vi "Configure.vi"(8 "error in (no error)":errorcluster, 11 "Template in":refnum<class "BMC.lvclass">) -> (0 "error out":errorcluster, 2 "cancelled?":bool, 3 "Template out":refnum<class "BMC.lvclass">)   [LabVIEW 2012, in "BMC.lvclass"]
doc: "The configure method configures the details for the RabbitMQ connection. \n\nIn the derived class, make a call to the parent for setting these parameters."
uses:
  BMC.lvclass
  <vilib>/Utility/miscctls.llb/LVPointTypeDef.ctl
  BMC.lvclass/BMC.ctl
  <vilib>/Distrio/Murmex/Murmex/Murmex.lvclass
panel:
  in  "Mapping file":path=path "D:/CLSM_Project/BMC/MultiMap.txt"
  in  "Flat mirror file":path=path "D:/CLSM_Project/BMC/zerovolt.txt"
  in  "button:call parent":bool
  in  "button:ok":bool
  in  "button:cancel":bool
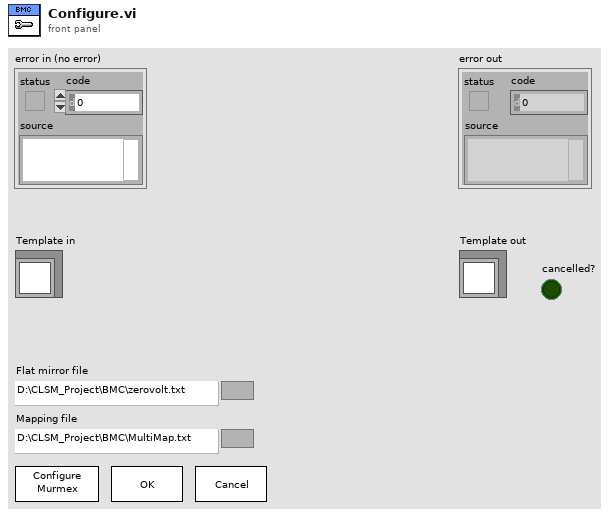
[diagram p1: front panel]
types:
  T1 = typedef "LVPointTypeDef.ctl" = cluster{"Horizontal":i16, "Vertical":i16}
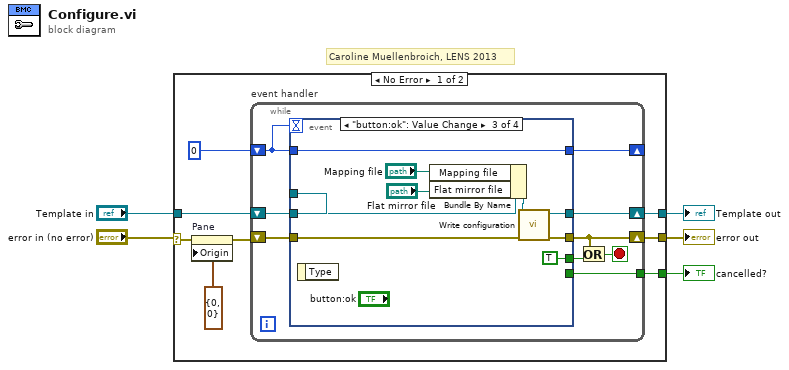
[diagram p0: block diagram]
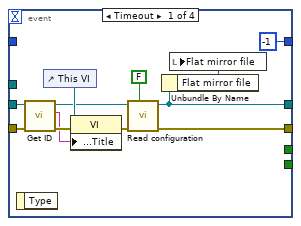
[diagram p2: hidden frame]
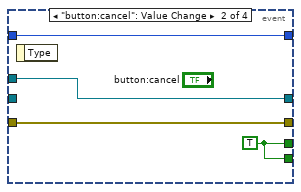
[diagram p3: hidden frame]
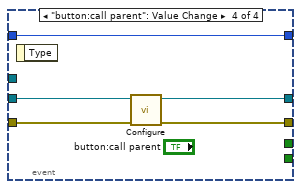
[diagram p4: hidden frame]
diagram:
  # "Caroline Muellenbroich, LENS 2013"
  n1 = case shown="No Error" "error in (no error)" {
    selector: "error in (no error)" -> [w7 w53]
    tunnel: [w13 w53] -> w5
    tunnel: [w12 _] -> w4
    tunnel: [w11 w54] -> w3
    tunnel: "Template in" -> [w10 w54]
    frame No Error {
      n2 = property on="Pane" class="Pane"(error in=w7, "Origin"=T1 {"Horizontal"=0, "Vertical"=0}) -> (error out=w6:errorcluster)  [unwired: 1 in, 1 out]
      n3 = while "event handler" {
        tunnel: [w22] -> w12
        shift-right: [w21] -> w11
        shift-left: w10 -> [w19]
        shift-right: [w18] -> w13
        shift-left: w6 -> [w20]
        shift-right: [w15] -> _
        shift-left: 0 -> [w14]
        stop <- w16 stop-if-true
        n4 = event shown="[2] \"button:ok\": Value Change" {
          selector: _ -> [_ _ _ _]
          dyn-events: _ -> [_ _ _ _]
          timeout: w14 -> [_ _ _ _]
          tunnel: [w34 w37 w42 w50] -> w18
          tunnel: [_ w36 _ _] -> w22
          tunnel: [w33 w38 w44 w49] -> w21
          tunnel: w20 -> [w26 w37 w43 w51]
          tunnel: w19 -> [w25 _ w46 w52]
          tunnel: w19 -> [_ w38 _ _]
          tunnel: [_ w36 TRUE ("cancelled?") _] -> w17
          tunnel: [-1 w35 w41 w48] -> w15
          tunnel: w14 -> [_ w35 w41 w48]
          event Timeout {
            n5 = event-data() -> ()  [unwired: 1 in, 1 out]
            n6 = call <vilib>:"Get ID.vi"("error in (no error)"=w26, "Murmex in"=w25) -> ("error out"=w30:errorcluster, "component id"=w28:string, "Murmex out"=w24:refnum<class "BMC.lvclass">)  [unwired: 7 in]
            n7 = control-ref of="This VI"() -> (w29:refnum<vi>)
            n8 = property class="VI"(reference=w29, error in=w30, "Front Panel.Title"=w28) -> (error out=w27:errorcluster)  [unwired: 1 out]
            n9 = call-dynamic "Read configuration.vi"("force loading?"=FALSE, "error in (no error)"=w27, "Template in"=w24) -> ("error out"=w34:errorcluster, "Template out"=w33:refnum<class "BMC.lvclass">)  [unwired: 7 in]
            n10 = Unbundle By Name(w33) -> ("Flat mirror file"=w32:path)
            n11 = local write "Flat mirror file"(w32) -> ()
          }
          event "button:cancel": Value Change {
            w36 = TRUE ("cancelled?")
            n12 = event-data() -> ()  [unwired: 1 in, 1 out]
          }
          event "button:ok": Value Change {
            n13 = event-data() -> ()  [unwired: 1 in, 1 out]
            n14 = Bundle By Name(cluster=w46, "Mapping file"="Mapping file", "Flat mirror file"="Flat mirror file") -> (w45:refnum<class "BMC.lvclass">)
            n15 = call-dynamic "Write configuration.vi"("error in (no error)"=w43, "Template in"=w45) -> ("error out"=w42:errorcluster, "Template out"=w44:refnum<class "BMC.lvclass">)  [unwired: 8 in]
          }
          event "button:call parent": Value Change {
            n16 = event-data() -> ()  [unwired: 1 in, 1 out]
            n17 = call-parent "Configure.vi"("error in (no error)"=w51, "Murmex in"=w52) -> ("error out"=w50:errorcluster, "Murmex out"=w49:refnum<class "BMC.lvclass">)  [unwired: 7 in, 1 out]
          }
        }
        n18 = Or(x=w18, y=w17) -> (x .or. y?=w16:bool)
      }
    }
    frame Error {
    }
  }
  "error out" <- w5
  "Template out" <- w3
  "cancelled?" <- w4
